vi "SPL2Phon.vi"(9 "Phone Precision in":dbl=10.0, 10 "SPL in":dbl[](array[numeric]), 11 "Frequency in":dbl[](array[numeric])) -> (3 "Phon out":dbl[](array[numeric]))   [LabVIEW 2013]
panel:
  out "XY Graph 3":cluster{"Frequency":dbl[], "SPL":dbl[]}[](graph)
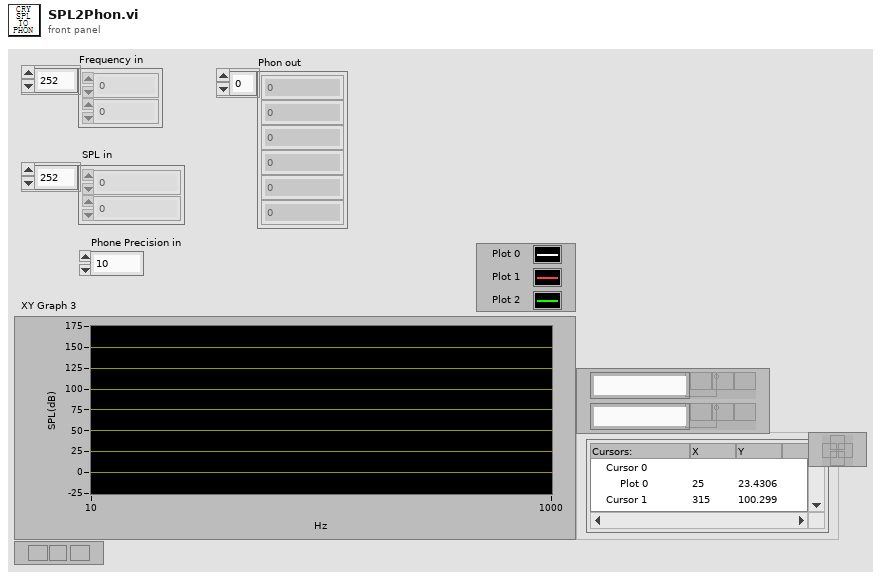
[diagram p1: front panel]
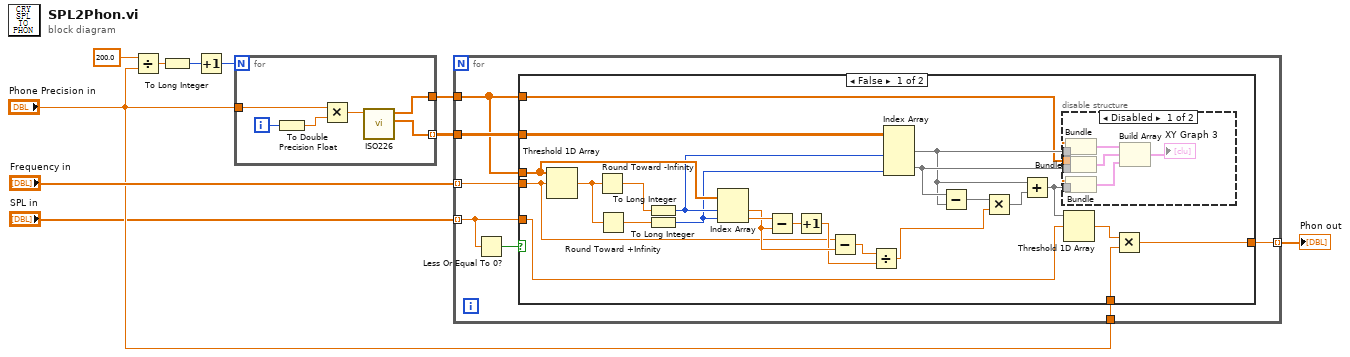
[diagram p0: block diagram]
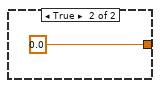
[diagram p3: hidden frame]
diagram:
  n1 = Divide(x=200.0, y="Phone Precision in") -> (x/y=w6:dbl)
  n2 = To Long Integer(number=w6) -> (32bit integer=w5:i32)
  n3 = Increment(x=w5) -> (x+1=w4:i32)
  n4 = for {
    N: w4 -> [_]
    tunnel: [w15] -> w1
    tunnel: [w13] -> w2 mode=indexing
    tunnel: "Phone Precision in" -> [w11]
    i -> [w16]
    n5 = To Double Precision Float(number=w16) -> (double precision float=w12:dbl)
    n6 = Multiply(x=w11, y=w12) -> (x*y=w14:dbl)
    n7 = call "ISO226.vi"("Phone number"=w14) -> ("SPL"=w13:dbl[], "Frequency"=w15:dbl[])  [unwired: 9 in]
  }
  n8 = for {
    tunnel: "Frequency in" -> [w22] mode=indexing
    tunnel: w2 -> [w23]
    tunnel: w1 -> [w17]
    tunnel: "SPL in" -> [w19] mode=indexing
    tunnel: "Phone Precision in" -> [w21]
    tunnel: [w20] -> w8 mode=indexing
    n9 = Less Or Equal To 0?(x=w19) -> (x <= 0?=w18:bool)
    n10 = case shown="False" w18 {
      tunnel: w17 -> [w45 _]
      tunnel: w23 -> [w38 _]
      tunnel: w17 -> [w30 _]
      tunnel: w22 -> [w28 _]
      tunnel: w19 -> [w27 _]
      tunnel: w21 -> [w25 _]
      tunnel: [w24 0.0] -> w20
      frame False {
        n11 = Threshold 1D Array(2:w28, 3:w45) -> (0:w47:dbl)  [unwired: 1 in]
        n12 = Round Toward -Infinity(1:w47) -> (0:w46:dbl)
        n13 = Round Toward +Infinity(x=w47) -> (ceil(x): smallest int >= x=w44:dbl)
        n14 = To Long Integer(number=w46) -> (32bit integer=w37:i32)
        n15 = To Long Integer(number=w44) -> (32bit integer=w36:i32)
        n16 = Index Array(array=w45, index #1=w37, index #2=w36) -> (element #1=w40:dbl, element #2=w41:dbl)
        n17 = Subtract(x=w41, y=w40) -> (x-y=w43:dbl)
        n18 = Increment(x=w43) -> (x+1=w39:dbl)
        n19 = Subtract(x=w28, y=w40) -> (x-y=w42:dbl)
        n20 = Divide(x=w42, y=w39) -> (x/y=w32:dbl)
        n21 = Index Array(array=w38, index (col) #1=w37, index (col) #2=w36) -> (element #1=w31:dbl[], element #2=w35:dbl[])  [unwired: 2 in]
        n22 = Subtract(x=w35, y=w31) -> (x-y=w33:dbl[])
        n23 = Multiply(x=w33, y=w32) -> (x*y=w34:dbl[])
        n24 = Add(x=w31, y=w34) -> (x+y=w29:dbl[])
        n25 = disable-structure shown="Disabled" {
          disable-tunnel: w35 -> [w52 _]
          disable-tunnel: w31 -> [w51 _]
          disable-tunnel: w30 -> [w50 _]
          disable-tunnel: w29 -> [w48 _]
          frame Disabled {
            n26 = Bundle("Frequency"=w50, "SPL"=w51) -> (w55:cluster{"Frequency":dbl[], "SPL":dbl[]})  [unwired: 1 in]
            n27 = Bundle("Frequency"=w50, "SPL"=w52) -> (w54:cluster{"Frequency":dbl[], "SPL":dbl[]})  [unwired: 1 in]
            n28 = Bundle("Frequency"=w50, w48) -> (w49:cluster{"Frequency":dbl[], dbl[]})  [unwired: 1 in]
            n29 = Build Array(w55, w54, w49) -> (→"XY Graph 3":cluster{"Frequency":dbl[], "SPL":dbl[]}[])
          }
          frame Enabled {
          }
        }
        n30 = Threshold 1D Array(2:w27, 3:w29) -> (0:w26:dbl)  [unwired: 1 in]
        n31 = Multiply(x=w26, y=w25) -> (x*y=w24:dbl)
      }
      frame True {
      }
    }
  }
  "Phon out" <- w8
